vi "TracesCreate.vi"(6 "PixmapWrite error":errorcluster, 10 "Traces.txt path":path) -> (4 "TracesCreate error":errorcluster)   [LabVIEW 2023]
uses:
  <vilib>/Utility/error.llb/Trim Whitespace One-Sided.vi
panel:
  in  "User interface":T1(tab)
  in  "User entries":enum32{""}(tab)
  in  "Customization":enum32{"Customization"}(tab)
  in  "Colors":enum32{"Colors"}(tab)
  in  "Size":enum32{"Size"}(tab)
  out "Traces.txt":string
  in  "Loop FOR 1":enum32{"Loop FOR 1"}(tab)
  in  "Arrays":enum32{"Arrays"}(tab)
  in  "Script.m":enum32{"Script.m"}(tab)
  in  "Extract.c output string scan":enum32{"Extract.c output string scan"}(tab)
  in  "T: tt1 tt2 tt3 ...":enum32{"T: tt1 tt2 tt3 ..."}(tab)
  in  "C: cc":enum32{"C: cc"}(tab)
  in  "Loop FOR 2":enum32{"Loop FOR 2"}(tab)
  in  "LabVIEW":enum32{"LabVIEW"}(tab)
  in  "MATLAB":enum32{"MATLAB"}(tab)
  in  "C":enum32{"C"}(tab)
  in  "MATLAB":enum32{"MATLAB"}(tab)
  in  "C":enum32{"C"}(tab)
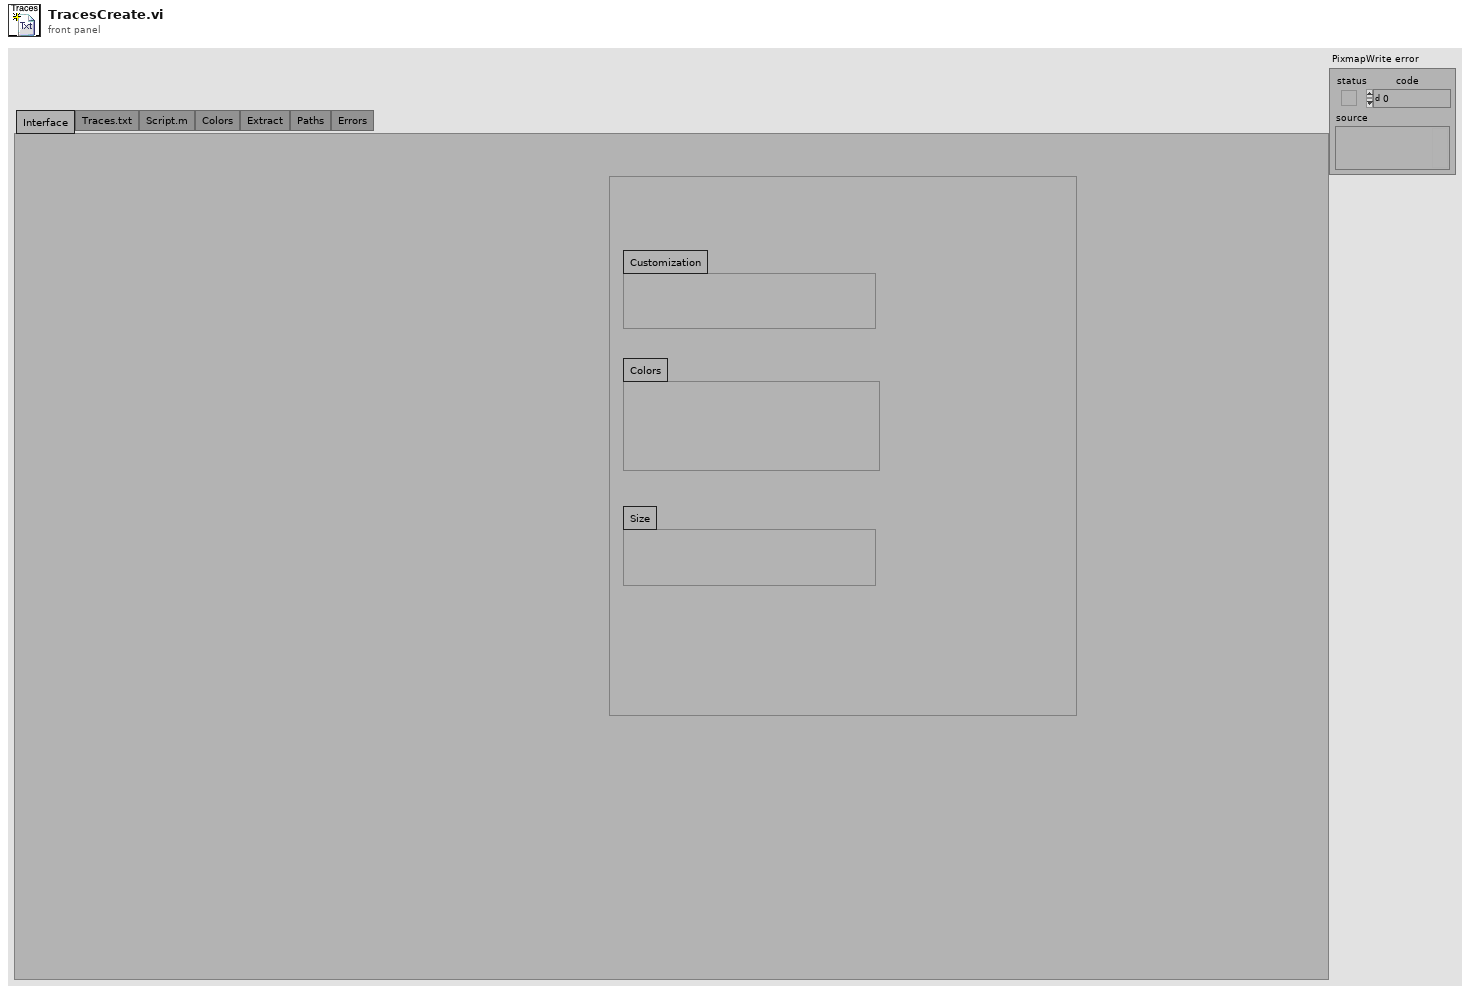
[diagram p1: front panel]
types:
  T1 = enum32{"Interface", "Traces.txt", "Script.m", "Colors", "Extract", "Paths", "Errors"}
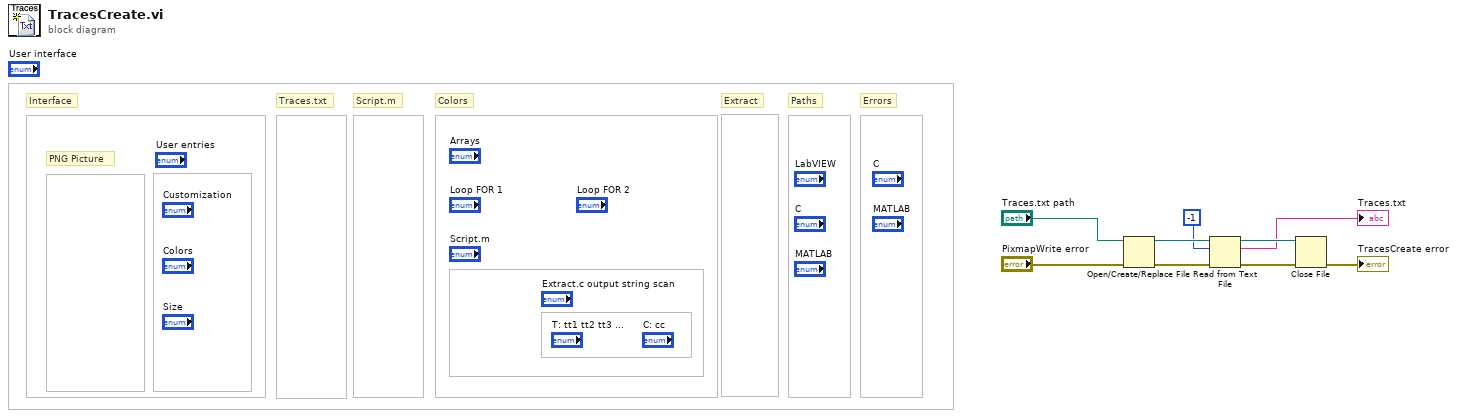
[diagram p0: block diagram]
diagram:
  # "PNG Picture"
  # "Errors"
  # "Paths"
  # "Extract"
  # "Colors"
  # "Script.m"
  # "Traces.txt"
  # "Interface"
  n1 = Open/Create/Replace File(file path (use dialog)="Traces.txt path", error in="PixmapWrite error") -> (refnum out=w7:refnum<file>, error out=w9:errorcluster)  [unwired: 4 in, 1 out]
  n2 = Read from Text File(file (use dialog)=w7, count=-1, error in=w9) -> (refnum out=w5:refnum<file>, text=→"Traces.txt":string, error out=w8:errorcluster)  [unwired: 1 in, 1 out]
  n3 = Close File(refnum=w5, error in=w8) -> (error out=→"TracesCreate error":errorcluster)  [unwired: 1 out]
